vi "Get GUI Control Builder Director.vi"(8 "error in (no error)":errorcluster, 11 "Panel Control_Ref in":refnum<class "Panel Controller.lvclass">) -> (0 "error out":errorcluster, 2 "GUI Control Builder Director.lvclass":refnum<class "GUI Control Builder Director.lvclass">, 3 "Panel Control_Ref out":refnum<class "Panel Controller.lvclass">)   [LabVIEW 2015, in "Panel Controller.lvclass"]
uses:
  Panel Controller.lvclass
  GUI/GUI Builder Director/GUI Control Builder Director.lvclass
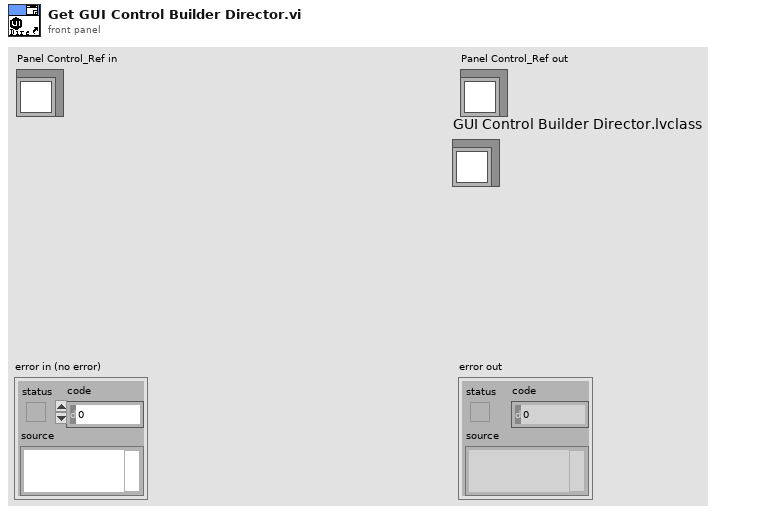
[diagram p1: front panel]
types:
  T1 = typedef "Panel Controller.lvclass/ObjectAttributes.ctl" = cluster{"Sub Panel Ref":refnum<vi>, "Panel_Q":refnum<queue>, "VI Running Refnum":refnum<vi>, "Brower Controller_Q":refnum<class "Message Enqueuer.lvclass">, "GUI Control Builder Director.lvclass":refnum<class "GUI Control Builder Director.lvclass">, "Panel GUI Manager.lvclass":refnum<class "Panel GUI Manager.lvclass">}
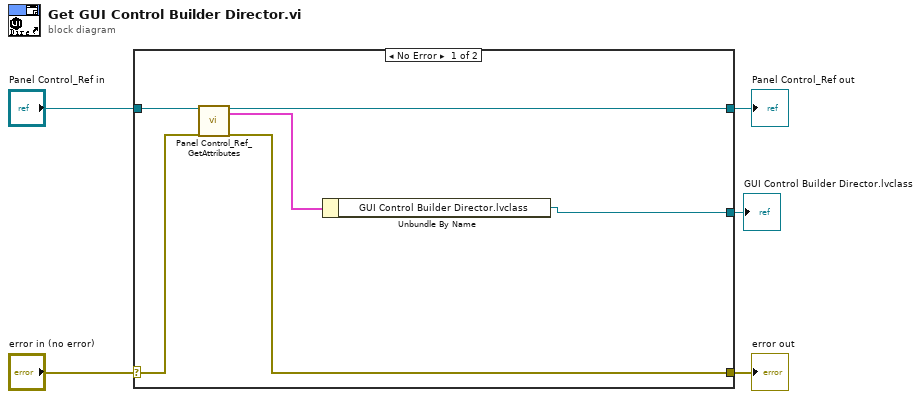
[diagram p0: block diagram]
diagram:
  n1 = case shown="No Error" "error in (no error)" {
    selector: "error in (no error)" -> [w10 w13]
    tunnel: [w9 w13] -> w4
    tunnel: [w6 w12] -> w2
    tunnel: "Panel Control_Ref in" -> [w11 w12]
    tunnel: [w7 _] -> w1
    frame No Error {
      n2 = call "Panel Control_Ref_GetAttributes.vi"("reference in"=w11, "error in (no error)"=w10) -> ("reference out"=w6:refnum<class "Panel Controller.lvclass">, "Data"=w8:T1, "error out"=w9:errorcluster)  [unwired: 14 in, 1 out]
      n3 = Unbundle By Name(w8) -> ("GUI Control Builder Director.lvclass"=w7:refnum<class "GUI Control Builder Director.lvclass">)
    }
    frame Error {
    }
  }
  "error out" <- w4
  "Panel Control_Ref out" <- w2
  "GUI Control Builder Director.lvclass" <- w1
